vi "Read_Path-to-logfile.vi"(8 "error in (no error)":errorcluster, 11 "StatusLog in":refnum<class "StatusLog.lvclass">) -> (0 "error out":errorcluster, 2 "Path to logfile":path, 3 "StatusLog out":refnum<class "StatusLog.lvclass">)   [LabVIEW 2018, in "StatusLog.lvclass"]
uses:
  StatusLog.lvclass
  StatusLog.lvclass/StatusLog.ctl
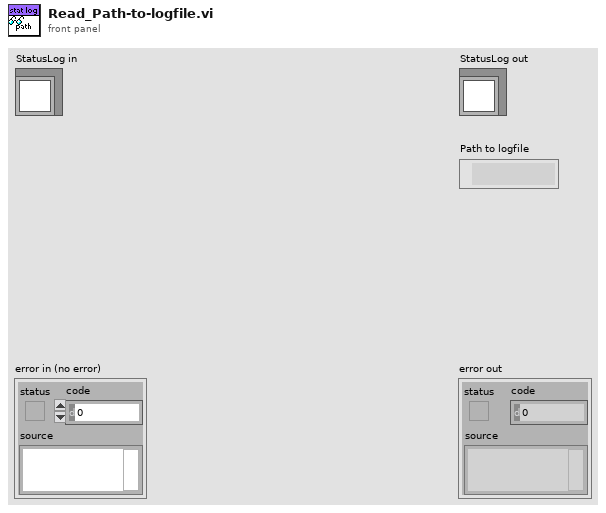
[diagram p1: front panel]
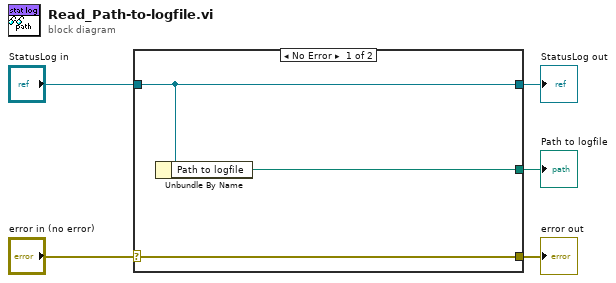
[diagram p0: block diagram]
diagram:
  n1 = case shown="No Error" "error in (no error)" {
    selector: "error in (no error)" -> [w8 w9]
    tunnel: [w8 w9] -> w4
    tunnel: [w7 w10] -> w2
    tunnel: "StatusLog in" -> [w7 w10]
    tunnel: [w6 _] -> w1
    frame No Error {
      n2 = Unbundle By Name(w7) -> ("Path to logfile"=w6:path)
    }
    frame Error {
    }
  }
  "error out" <- w4
  "StatusLog out" <- w2
  "Path to logfile" <- w1
